vi "ElapsedRT_us.vi"(11 "Error in":errorcluster caption="Error in (no error)", 12 "Start time in":i64=-1 caption="Start time in (-1: init) [µs]" min=-1 max=4294967295) -> (8 "Elapsed time":i32 caption="Elapsed time [µs]", 13 "Now":i64 caption="Now [µs]", 14 "Start time out":i64 caption="Start time out [µs]", 15 "Error out":errorcluster)   [LabVIEW 2017, in "GPTiming.lvlib"]
doc: "Calculates <B>Elapsed time</B> since <B>Start time in</B>.\n\n<B>Start time in</B> will be returned in <B>Start time out</B>. Set <B>Start time in</B> to -1 (or leave it unwired) to get the current time returned in <B>Start time out</B> instead. <B>Now</B> will always be the current time.\n\nThis VI uses the Real-Time microsecond tick counter and will be able to count for 2^31-1 microseconds (almost 36 minutes) before <B>Elapsed time</B> wraps around.\n\nThis VI is inlined. <B>Error in</B> is wired straight through to <B>Error out</B> to enable optional dataflow dependency (offering control of when <B>Now</B> is).\n\nSteen Schmidt\nGPower\n5/12 2013"
uses:
  GPTiming.lvlib
panel:
  # "Copyright © 2013\nGPower\nSee enclosed license file for terms and conditions"
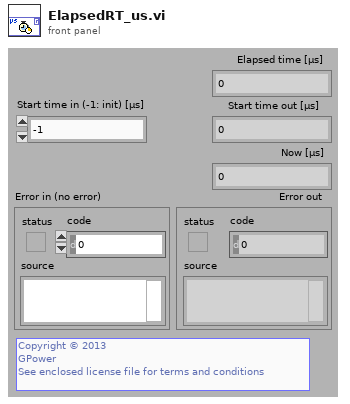
[diagram p1: front panel]
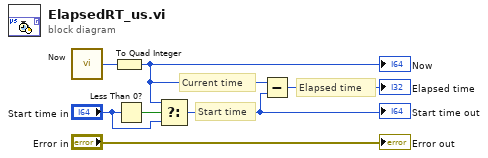
[diagram p0: block diagram]
diagram:
  # "Elapsed time"
  # "Current time"
  # "Start time"
  n1 = call "Now"() -> ("Tick Count(uSec)"=w1:u32)
  n2 = To Quad Integer(1:w1) -> (0:w2:i64)
  "Now" <- w2
  n3 = Less Than 0?(x="Start time in") -> (x < 0?=w7:bool)
  n4 = Select(t=w2, s=w7, f="Start time in") -> (s? t:f=w4:i64)
  "Start time out" <- w4
  n5 = Subtract(x=w2, y=w4) -> (x-y=→"Elapsed time":i64)
  "Error out" <- "Error in"
